vi "Scan_Table_Mode.vi"(0 "Mode":T1) -> (1 "Simulate Mode ?":bool, 2 "Log Full Res Data?":bool)   [LabVIEW 2015]
uses:
  Anemometry/Anemometry Sub Vis/Controls/Serveds.ctl
  Anemometry/Anemometry Sub Vis/Globals/Constants_global.vi
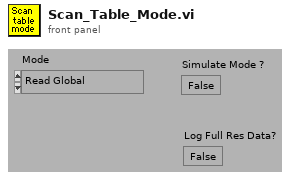
[diagram p1: front panel]
types:
  T1 = typedef "Serveds.ctl" = enum16{"Read Global", "Load Global From File"}
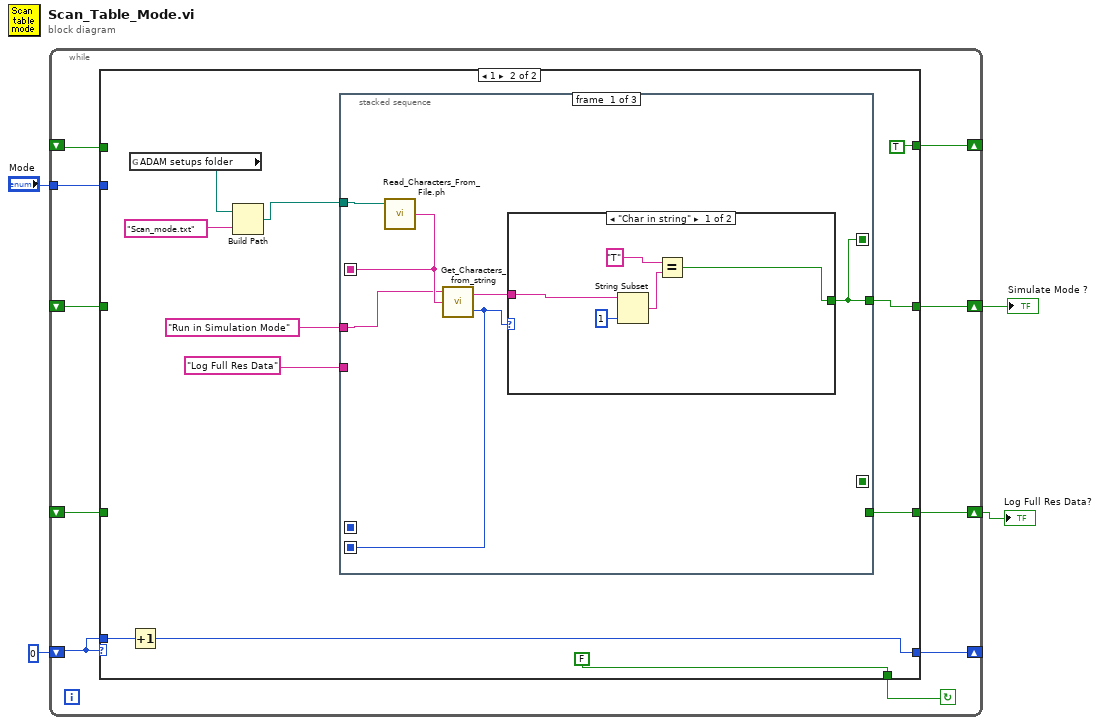
[diagram p0: block diagram]
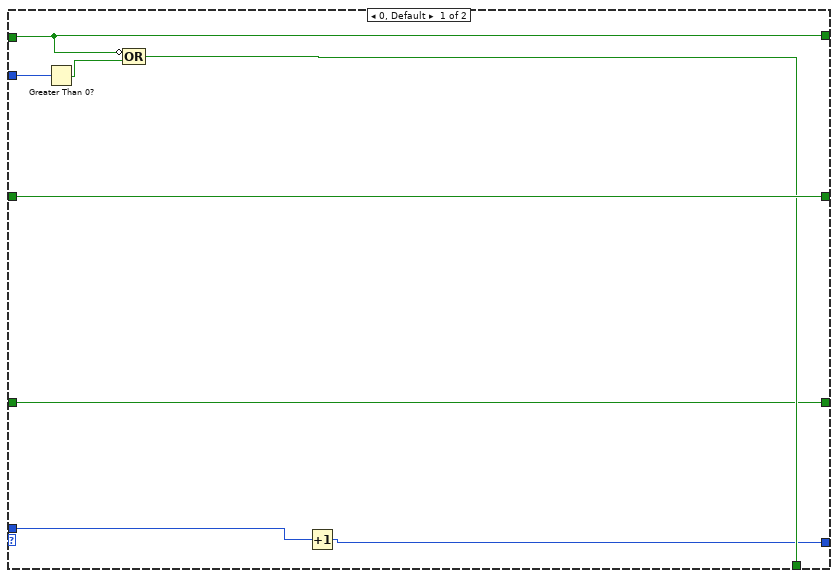
[diagram p2: hidden frame]
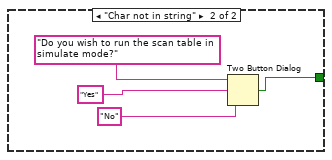
[diagram p3: hidden frame]
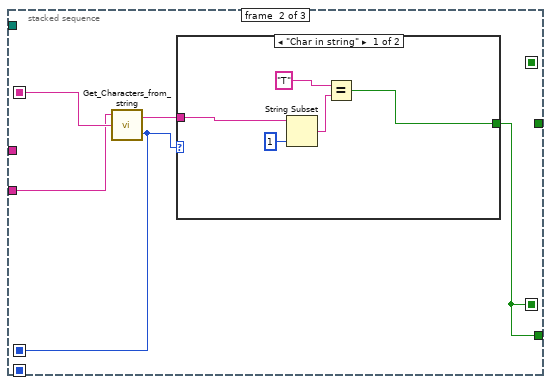
[diagram p4: hidden frame]
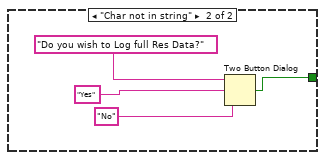
[diagram p5: hidden frame]
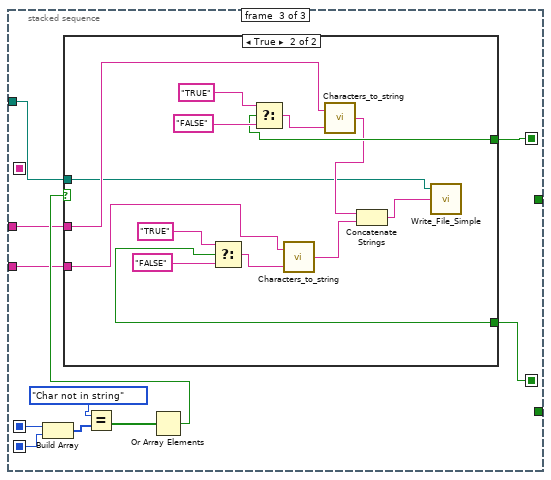
[diagram p6: hidden frame]
diagram:
  n1 = while {
    tunnel: "Mode" -> [w8]
    shift-left: 0 -> [w9]
    shift-right: [w11] -> _
    shift-left: _ -> [w13]
    shift-right: [w10] -> w2
    shift-left: _ -> [w14]
    shift-right: [w7] -> _
    shift-right: [w6] -> w1
    shift-left: _ -> [w5]
    stop <- w12 continue-if-true
    n2 = case shown="1" w9 {
      tunnel: w14 -> [w16 _]
      tunnel: w13 -> [w22 _]
      tunnel: [w19 FALSE] -> w12
      tunnel: [w17 w31] -> w11
      tunnel: [w22 w28] -> w10
      tunnel: w9 -> [w18 w32]
      tunnel: w8 -> [w21 _]
      tunnel: [w16 TRUE] -> w7
      tunnel: [w15 w23] -> w6
      tunnel: w5 -> [w15 _]
      frame 0, Default {
        n3 = Greater Than 0?(x=w21) -> (x > 0?=w20:bool)
        n4 = Compound Arithmetic op=OR(invert w16, w20) -> (w19:bool)
        n5 = Increment(x=w18) -> (x+1=w17:i32)
      }
      frame 1 {
        n6 = global read "Constants_global.vi" "ADAM setups folder"() -> (w30:path)
        n7 = Increment(x=w32) -> (x+1=w31:i32)
        n8 = Build Path(base path=w30, name or relative path="Scan_mode.txt" ("Substring")) -> (appended path=w26:path)
        n9 = stacked-sequence {
          seq-local: [w37 _ _] -> [_ w52 _]
          seq-local: [_ w50 _] -> [_ _ w72]
          seq-local: [w35 _ _] -> [_ _ w71]
          seq-local: [w34 _ _] -> [_ _ w67]
          seq-local: [_ w49 _] -> [_ _ w65]
          tunnel: "Run in Simulation Mode" ("character string") -> [w36 _ w66]
          tunnel: [w34 _ _] -> w28
          tunnel: [_ w49 _] -> w23
          tunnel: w26 -> [w38 _ w64]
          tunnel: "Log Full Res Data" ("character string") -> [_ w51 w63]
          frame #0 {
            n10 = call "Read_Characters_From_File.ph.vi"("file path (dialog if empty)"=w38) -> ("character string"=w37:string)  [unwired: 1 in, 7 out]
            n11 = call "Get_Characters_from_string.vi"("Input string"=w37, "Variable name"=w36) -> ("Status"=w35:enum16{"Char in string", "Char not in string"}, "Value"=w39:string)  [unwired: 1 in]
            n12 = case shown="\"Char in string\"" w35 {
              tunnel: w39 -> [w44 _]
              tunnel: [w40 w45] -> w34
              frame "Char in string" {
                n13 = String Subset(string=w44, length (rest)=1 ("length (rest)")) -> (substring=w42:string)  [unwired: 1 out]
                n14 = Equal?(x="T", y=w42) -> (x = y?=w40:bool)
              }
              frame "Char not in string" {
                n15 = Two Button Dialog(message="Do you wish to run the scan table in simulate mode?", 1:"No" ("F button name (\"Cancel\")"), 2:"Yes" ("T button name (\"OK\")")) -> (T button?=w45:bool)
              }
            }
          }
          frame #1 {
            n16 = call "Get_Characters_from_string.vi"("Input string"=w52, "Variable name"=w51) -> ("Status"=w50:enum16{"Char in string", "Char not in string"}, "Value"=w53:string)  [unwired: 1 in]
            n17 = case shown="\"Char in string\"" w50 {
              tunnel: w53 -> [w58 _]
              tunnel: [w54 w59] -> w49
              frame "Char in string" {
                n18 = String Subset(string=w58, length (rest)=1 ("length (rest)")) -> (substring=w56:string)  [unwired: 1 out]
                n19 = Equal?(x="T", y=w56) -> (x = y?=w54:bool)
              }
              frame "Char not in string" {
                n20 = Two Button Dialog(message="Do you wish to Log full Res Data?", 1:"No" ("F button name (\"Cancel\")"), 2:"Yes" ("T button name (\"OK\")")) -> (T button?=w59:bool)
              }
            }
          }
          frame #2 {
            n21 = Build Array(w72, w71) -> (w70:enum16{"Char in string", "Char not in string"}[])
            n22 = Equal?(x=enum16{"Char in string", "Char not in string"}."Char not in string" ("Status"), y=w70) -> (x = y?=w69:bool[])
            n23 = Or Array Elements(Boolean array=w69) -> (logical OR=w68:bool)
            n24 = case shown="True" w68 {
              tunnel: w67 -> [_ w84]
              tunnel: w66 -> [_ w83]
              tunnel: w65 -> [_ w79]
              tunnel: w63 -> [_ w78]
              tunnel: w64 -> [_ w74]
              frame False {
              }
              frame True {
                n25 = Select(t="TRUE" ("Characters to write"), s=w79, f="FALSE") -> (s? t:f=w80:string)
                n26 = Select(t="TRUE" ("Characters to write"), s=w84, f="FALSE") -> (s? t:f=w87:string)
                n27 = call "Characters_to_string.vi"("Characters to write"=w80, "Label for characters"=w78) -> ("Output string"=w76:string)
                n28 = call "Characters_to_string.vi"("Characters to write"=w87, "Label for characters"=w83) -> ("Output string"=w75:string)
                n29 = Concatenate Strings(w75, w76) -> (w77:string)
                n30 = call "Write_File_Simple.vi"("character string"=w77, "file path"=w74) -> ()  [unwired: 1 in, 2 out]
              }
            }
          }
        }
      }
    }
  }
  "Simulate Mode ?" <- w2
  "Log Full Res Data?" <- w1
